vi "Create Project Item - Root Project.vi"(8 "Error In":errorcluster, 11 "Project Reference":refnum<vi>) -> (0 "Error Out":errorcluster, 1 "project item":T1, 2 "Owned Items[]":refnum<vi>[](array[refnum]), 3 "Project Reference Out":refnum<vi>)   [LabVIEW 2014, in "i3-docs.lvlib"]
uses:
  i3-docs.lvlib
  Controls/project_item.ctl
  Controls/image_information.ctl
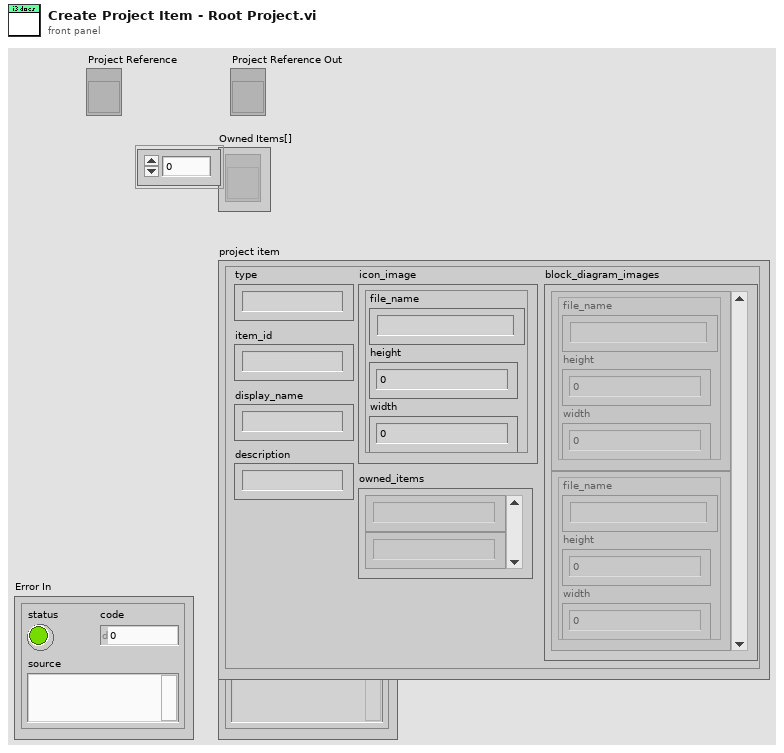
[diagram p1: front panel]
types:
  T1 = typedef "i3-docs.lvlib/project_item.ctl" = cluster{"type":string, "owned_items":string[], "item_id":string, "display_name":string, "description":string, "block_diagram_images":T2[], "icon_image":T2}
  T2 = typedef "i3-docs.lvlib/image_information.ctl" = cluster{"file_name":string, "height":i32, "width":i32}
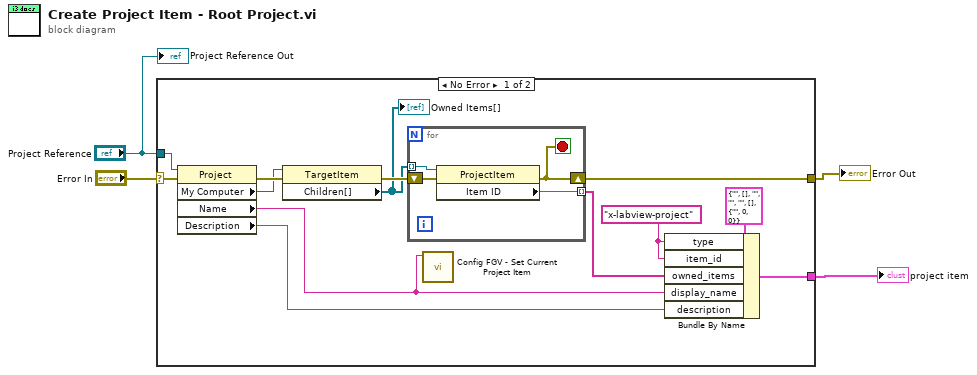
[diagram p0: block diagram]
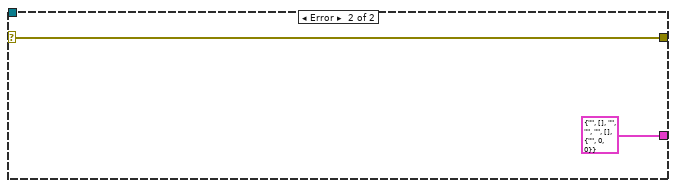
[diagram p2: hidden frame]
diagram:
  n1 = case shown="No Error" "Error In" {
    selector: "Error In" -> [w7 w23]
    tunnel: "Project Reference" -> [w9 _]
    tunnel: [w8 T1 {"type"="", "owned_items"=[], "item_id"="", "display_name"="", "description"="", "block_diagram_images"=[], "icon_image"={"file_name"="", "height"=0, "width"=0}} ("project_item")] -> w4
    tunnel: [w6 w23] -> w1
    frame No Error {
      w14 = "x-labview-project" ("type")
      n2 = property class="Project"(reference=w9, error in=w7) -> (error out=w17:errorcluster, "My Computer"=w16:refnum<vi>, "Name"=w5:string, "Description"=w13:string)  [unwired: 1 out]
      n3 = property class="TargetItem"(reference=w16, error in=w17) -> (error out=w12:errorcluster, "Children[]"=w11:refnum<vi>[])  [unwired: 1 out]
      "Owned Items[]" <- w11
      n4 = for {
        tunnel: w11 -> [w21] mode=indexing
        shift-right: [w19] -> w6
        shift-left: w12 -> [w20]
        tunnel: [w18] -> w10 mode=indexing
        stop <- w19 stop-if-true
        n5 = property class="ProjectItem"(reference=w21, error in=w20) -> (error out=w19:errorcluster, "Item ID"=w18:string)  [unwired: 1 out]
      }
      n6 = call "Config FGV - Set Current Project Item.vi"("Set Current Project Item"=w5) -> ()  [unwired: 11 in]
      n7 = Bundle By Name(cluster=T1 {"type"="", "owned_items"=[], "item_id"="", "display_name"="", "description"="", "block_diagram_images"=[], "icon_image"={"file_name"="", "height"=0, "width"=0}} ("project_item"), "type"=w14, "item_id"=w14, "owned_items"=w10, "display_name"=w5, "description"=w13) -> (w8:T1)
    }
    frame Error {
    }
  }
  "project item" <- w4
  "Error Out" <- w1
  "Project Reference Out" <- "Project Reference"
